vi "Poker Score.vi"(2 "Card Number":dbl) -> (0 "Poker Hands Score and Combination":T1(array[cluster]))   [LabVIEW 2014]
panel:
  in  "Pair's DBL":dbl
  in  "Pair's value":i32
  out "Score":dbl
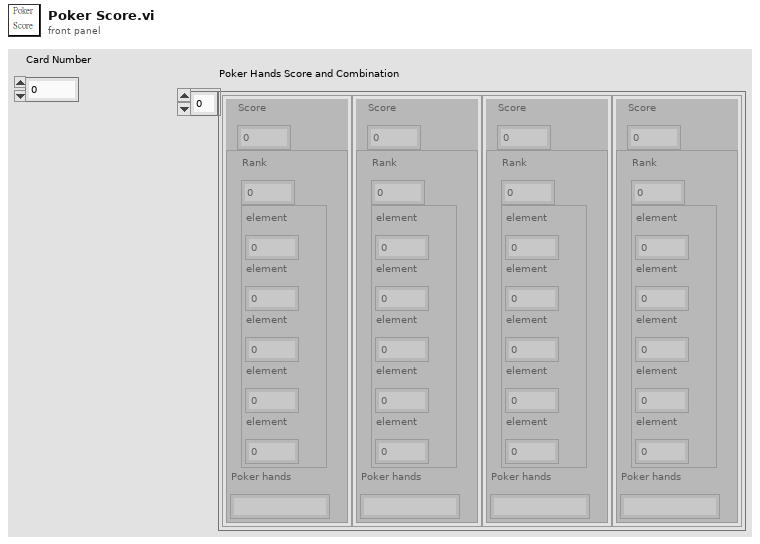
[diagram p1: front panel]
types:
  T1 = cluster{"Score":dbl, cluster{"Rank":i32, cluster{"element":dbl, "element":dbl, "element":dbl, "element":dbl, "element":dbl}, "Poker hands":string}}[]
  T2 = cluster{"Rank":i32, cluster{"element":dbl, "element":dbl, "element":dbl, "element":dbl, "element":dbl}, "Poker hands":string}[]
  T3 = cluster{"element":dbl, "element":dbl, "element":dbl, "element":dbl, "element":dbl}
  T4 = cluster{"Score":dbl, cluster{"Rank":i32, cluster{"element":dbl, "element":dbl, "element":dbl, "element":dbl, "element":dbl}, "Poker hands":string}}
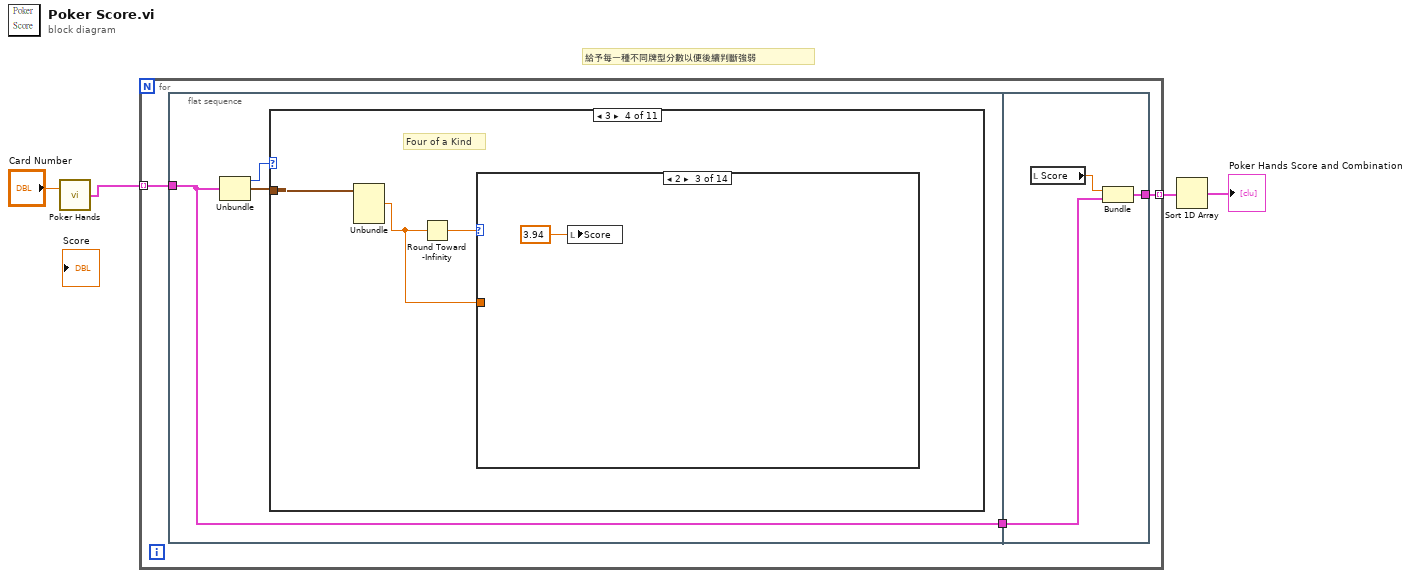
[diagram p0: block diagram]
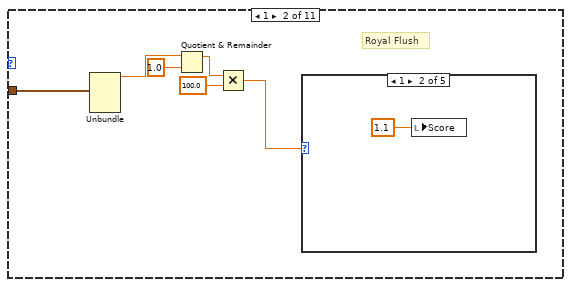
[diagram p3: hidden frame]
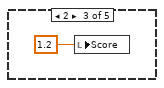
[diagram p5: hidden frame]
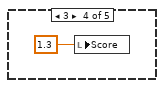
[diagram p6: hidden frame]
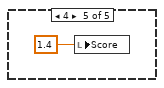
[diagram p7: hidden frame]
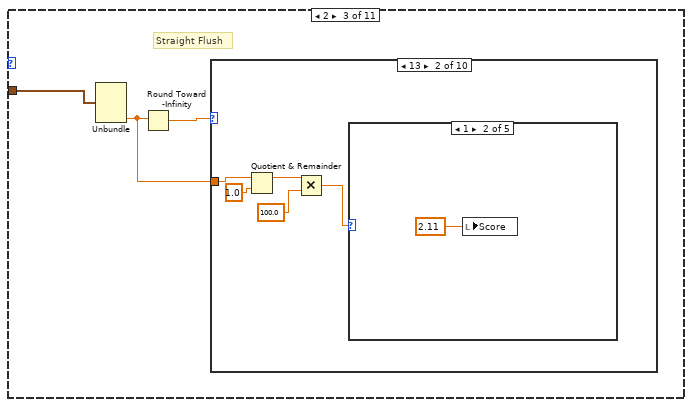
[diagram p8: hidden frame]
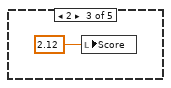
[diagram p11: hidden frame]
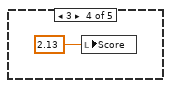
[diagram p12: hidden frame]
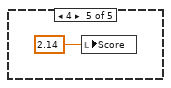
[diagram p13: hidden frame]
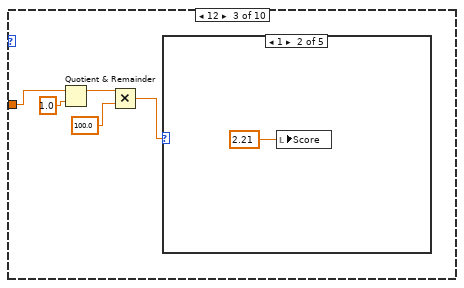
[diagram p14: hidden frame]
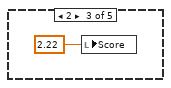
[diagram p16: hidden frame]
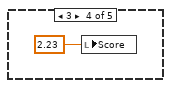
[diagram p17: hidden frame]
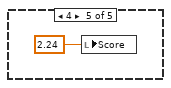
[diagram p18: hidden frame]
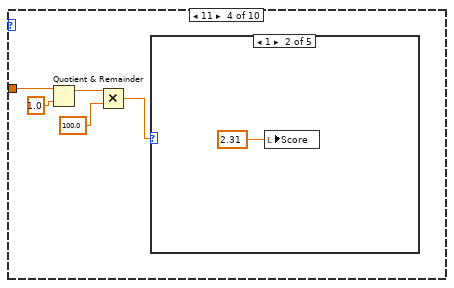
[diagram p19: hidden frame]
diagram:
  # "給予每一種不同牌型分數以便後續判斷強弱"
  n1 = call "Poker Hands.vi"("Card Number"="Card Number") -> ("Poker hands Rank and Combination"=w3:T2)  [unwired: 1 in]
  n2 = for {
    tunnel: w3 -> [w7] mode=indexing
    tunnel: [w5] -> w2 mode=indexing
    n3 = flat-sequence {
      tunnel: [w8] -> w6
      tunnel: w7 -> [w8]
      tunnel: w6 -> [w888]
      tunnel: [w887] -> w5
      frame #0 {
        n4 = Unbundle(w8) -> ("Rank"=w10:i32, w9:T3)  [unwired: 1 out]
        n5 = case shown="3" w10 {
          tunnel: w9 -> [_ w14 w23 w107 w123 w247 w322 w420 w555 w664 w808]
          frame 0, Default {
          }
          frame 1 {
            # "Royal Flush"
            n6 = Unbundle(w14) -> ("element"=w16:dbl)  [unwired: 4 out]
            n7 = Quotient & Remainder(x=w16, y=1.0) -> (x-y*floor(x/y)=w13:dbl)  [unwired: 1 out]
            n8 = Multiply(x=w13, y=100.0) -> (x*y=w11:dbl)
            n9 = case shown="1" w11 {
              frame 0, Default {
              }
              frame 1 {
                n10 = local write "Score"(1.1 ("Numeric")) -> ()
              }
              frame 2 {
                n11 = local write "Score"(1.2 ("Numeric")) -> ()
              }
              frame 3 {
                n12 = local write "Score"(1.3 ("Numeric")) -> ()
              }
              frame 4 {
                n13 = local write "Score"(1.4 ("Numeric")) -> ()
              }
            }
          }
          frame 2 {
            # "Straight Flush"
            n14 = Unbundle(w23) -> ("element"=w21:dbl)  [unwired: 4 out]
            n15 = Round Toward -Infinity(1:w21) -> (0:w22:dbl)
            n16 = case shown="13" w22 {
              tunnel: w21 -> [_ w28 w33 w42 w51 w60 w69 w78 w87 w96]
              frame 0, Default {
              }
              frame 13 {
                n17 = Quotient & Remainder(x=w28, y=1.0) -> (x-y*floor(x/y)=w26:dbl)  [unwired: 1 out]
                n18 = Multiply(x=w26, y=100.0) -> (x*y=w24:dbl)
                n19 = case shown="1" w24 {
                  frame 0, Default {
                  }
                  frame 1 {
                    n20 = local write "Score"(2.11 ("Numeric")) -> ()
                  }
                  frame 2 {
                    n21 = local write "Score"(2.12 ("Numeric")) -> ()
                  }
                  frame 3 {
                    n22 = local write "Score"(2.13 ("Numeric")) -> ()
                  }
                  frame 4 {
                    n23 = local write "Score"(2.14 ("Numeric")) -> ()
                  }
                }
              }
              frame 12 {
                n24 = Quotient & Remainder(x=w33, y=1.0) -> (x-y*floor(x/y)=w36:dbl)  [unwired: 1 out]
                n25 = Multiply(x=w36, y=100.0) -> (x*y=w34:dbl)
                n26 = case shown="1" w34 {
                  frame 0, Default {
                  }
                  frame 1 {
                    n27 = local write "Score"(2.21 ("Numeric")) -> ()
                  }
                  frame 2 {
                    n28 = local write "Score"(2.22 ("Numeric")) -> ()
                  }
                  frame 3 {
                    n29 = local write "Score"(2.23 ("Numeric")) -> ()
                  }
                  frame 4 {
                    n30 = local write "Score"(2.24 ("Numeric")) -> ()
                  }
                }
              }
              frame 11 {
                n31 = Quotient & Remainder(x=w42, y=1.0) -> (x-y*floor(x/y)=w45:dbl)  [unwired: 1 out]
                n32 = Multiply(x=w45, y=100.0) -> (x*y=w43:dbl)
                n33 = case shown="1" w43 {
                  frame 0, Default {
                  }
                  frame 1 {
                    n34 = local write "Score"(2.31 ("Numeric")) -> ()
                  }
                  frame 2 {
                    n35 = local write "Score"(2.32 ("Numeric")) -> ()
                  }
                  frame 3 {
                    n36 = local write "Score"(2.33 ("Numeric")) -> ()
                  }
                  frame 4 {
                    n37 = local write "Score"(2.34 ("Numeric")) -> ()
                  }
                }
              }
              frame 10 {
                n38 = Quotient & Remainder(x=w51, y=1.0) -> (x-y*floor(x/y)=w54:dbl)  [unwired: 1 out]
                n39 = Multiply(x=w54, y=100.0) -> (x*y=w52:dbl)
                n40 = case shown="1" w52 {
                  frame 0, Default {
                  }
                  frame 1 {
                    n41 = local write "Score"(2.41 ("Numeric")) -> ()
                  }
                  frame 2 {
                    n42 = local write "Score"(2.42 ("Numeric")) -> ()
                  }
                  frame 3 {
                    n43 = local write "Score"(2.43 ("Numeric")) -> ()
                  }
                  frame 4 {
                    n44 = local write "Score"(2.44 ("Numeric")) -> ()
                  }
                }
              }
              frame 9 {
                n45 = Quotient & Remainder(x=w60, y=1.0) -> (x-y*floor(x/y)=w63:dbl)  [unwired: 1 out]
                n46 = Multiply(x=w63, y=100.0) -> (x*y=w61:dbl)
                n47 = case shown="1" w61 {
                  frame 0, Default {
                  }
                  frame 1 {
                    n48 = local write "Score"(2.51 ("Numeric")) -> ()
                  }
                  frame 2 {
                    n49 = local write "Score"(2.52 ("Numeric")) -> ()
                  }
                  frame 3 {
                    n50 = local write "Score"(2.53 ("Numeric")) -> ()
                  }
                  frame 4 {
                    n51 = local write "Score"(2.54 ("Numeric")) -> ()
                  }
                }
              }
              frame 8 {
                n52 = Quotient & Remainder(x=w69, y=1.0) -> (x-y*floor(x/y)=w72:dbl)  [unwired: 1 out]
                n53 = Multiply(x=w72, y=100.0) -> (x*y=w70:dbl)
                n54 = case shown="1" w70 {
                  frame 0, Default {
                  }
                  frame 1 {
                    n55 = local write "Score"(2.61 ("Numeric")) -> ()
                  }
                  frame 2 {
                    n56 = local write "Score"(2.62 ("Numeric")) -> ()
                  }
                  frame 3 {
                    n57 = local write "Score"(2.63 ("Numeric")) -> ()
                  }
                  frame 4 {
                    n58 = local write "Score"(2.64 ("Numeric")) -> ()
                  }
                }
              }
              frame 7 {
                n59 = Quotient & Remainder(x=w78, y=1.0) -> (x-y*floor(x/y)=w81:dbl)  [unwired: 1 out]
                n60 = Multiply(x=w81, y=100.0) -> (x*y=w79:dbl)
                n61 = case shown="1" w79 {
                  frame 0, Default {
                  }
                  frame 1 {
                    n62 = local write "Score"(2.71 ("Numeric")) -> ()
                  }
                  frame 2 {
                    n63 = local write "Score"(2.72 ("Numeric")) -> ()
                  }
                  frame 3 {
                    n64 = local write "Score"(2.73 ("Numeric")) -> ()
                  }
                  frame 4 {
                    n65 = local write "Score"(2.74 ("Numeric")) -> ()
                  }
                }
              }
              frame 6 {
                n66 = Quotient & Remainder(x=w87, y=1.0) -> (x-y*floor(x/y)=w90:dbl)  [unwired: 1 out]
                n67 = Multiply(x=w90, y=100.0) -> (x*y=w88:dbl)
                n68 = case shown="1" w88 {
                  frame 0, Default {
                  }
                  frame 1 {
                    n69 = local write "Score"(2.81 ("Numeric")) -> ()
                  }
                  frame 2 {
                    n70 = local write "Score"(2.82 ("Numeric")) -> ()
                  }
                  frame 3 {
                    n71 = local write "Score"(2.83 ("Numeric")) -> ()
                  }
                  frame 4 {
                    n72 = local write "Score"(2.84 ("Numeric")) -> ()
                  }
                }
              }
              frame 5 {
                n73 = Quotient & Remainder(x=w96, y=1.0) -> (x-y*floor(x/y)=w99:dbl)  [unwired: 1 out]
                n74 = Multiply(x=w99, y=100.0) -> (x*y=w97:dbl)
                n75 = case shown="1" w97 {
                  frame 0, Default {
                  }
                  frame 1 {
                    n76 = local write "Score"(2.91 ("Numeric")) -> ()
                  }
                  frame 2 {
                    n77 = local write "Score"(2.92 ("Numeric")) -> ()
                  }
                  frame 3 {
                    n78 = local write "Score"(2.93 ("Numeric")) -> ()
                  }
                  frame 4 {
                    n79 = local write "Score"(2.94 ("Numeric")) -> ()
                  }
                }
              }
            }
          }
          frame 3 {
            # "Four of a Kind"
            n80 = Unbundle(w107) -> ("element"=w105:dbl)  [unwired: 4 out]
            n81 = Round Toward -Infinity(1:w105) -> (0:w106:dbl)
            n82 = case shown="2" w106 {
              tunnel: w105 -> [_ _ _ _ _ _ _ _ _ _ _ _ _ _]
              frame 0, Default {
              }
              frame 1 {
                n83 = local write "Score"(3.1 ("Numeric")) -> ()
              }
              frame 2 {
                n84 = local write "Score"(3.94 ("Numeric")) -> ()
              }
              frame 3 {
                n85 = local write "Score"(3.93 ("Numeric")) -> ()
              }
              frame 4 {
                n86 = local write "Score"(3.92 ("Numeric")) -> ()
              }
              frame 5 {
                n87 = local write "Score"(3.91 ("Numeric")) -> ()
              }
              frame 6 {
                n88 = local write "Score"(3.9 ("Numeric")) -> ()
              }
              frame 7 {
                n89 = local write "Score"(3.8 ("Numeric")) -> ()
              }
              frame 8 {
                n90 = local write "Score"(3.7 ("Numeric")) -> ()
              }
              frame 9 {
                n91 = local write "Score"(3.6 ("Numeric")) -> ()
              }
              frame 10 {
                n92 = local write "Score"(3.5 ("Numeric")) -> ()
              }
              frame 11 {
                n93 = local write "Score"(3.4 ("Numeric")) -> ()
              }
              frame 12 {
                n94 = local write "Score"(3.3 ("Numeric")) -> ()
              }
              frame 13 {
                n95 = local write "Score"(3.2 ("Numeric")) -> ()
              }
            }
          }
          frame 4 {
            # "Full House"
            n96 = Unbundle(w123) -> ("element"=w121:dbl)  [unwired: 4 out]
            n97 = Round Toward -Infinity(1:w121) -> (0:w122:dbl)
            n98 = case shown="1" w122 {
              tunnel: w121 -> [_ w124 w133 w142 w151 w160 w169 w178 w187 w196 w205 w214 w223 w232]
              frame 0, Default {
              }
              frame 1 {
                n99 = Quotient & Remainder(x=w124, y=1.0) -> (x-y*floor(x/y)=w127:dbl)  [unwired: 1 out]
                n100 = Multiply(x=w127, y=100.0) -> (x*y=w125:dbl)
                n101 = case shown="1" w125 {
                  frame 0, Default {
                  }
                  frame 1 {
                    n102 = local write "Score"(4.11 ("Numeric")) -> ()
                  }
                  frame 2 {
                    n103 = local write "Score"(4.12 ("Numeric")) -> ()
                  }
                  frame 3 {
                    n104 = local write "Score"(4.13 ("Numeric")) -> ()
                  }
                  frame 4 {
                    n105 = local write "Score"(4.14 ("Numeric")) -> ()
                  }
                }
              }
              frame 2 {
                n106 = Quotient & Remainder(x=w133, y=1.0) -> (x-y*floor(x/y)=w136:dbl)  [unwired: 1 out]
                n107 = Multiply(x=w136, y=100.0) -> (x*y=w134:dbl)
                n108 = case shown="4" w134 {
                  frame 0, Default {
                  }
                  frame 1 {
                    n109 = local write "Score"(4.981 ("Numeric")) -> ()
                  }
                  frame 2 {
                    n110 = local write "Score"(4.982 ("Numeric")) -> ()
                  }
                  frame 3 {
                    n111 = local write "Score"(4.983 ("Numeric")) -> ()
                  }
                  frame 4 {
                    n112 = local write "Score"(4.984 ("Numeric")) -> ()
                  }
                }
              }
              frame 3 {
                n113 = Quotient & Remainder(x=w142, y=1.0) -> (x-y*floor(x/y)=w145:dbl)  [unwired: 1 out]
                n114 = Multiply(x=w145, y=100.0) -> (x*y=w143:dbl)
                n115 = case shown="4" w143 {
                  frame 0, Default {
                  }
                  frame 1 {
                    n116 = local write "Score"(4.971 ("Numeric")) -> ()
                  }
                  frame 2 {
                    n117 = local write "Score"(4.972 ("Numeric")) -> ()
                  }
                  frame 3 {
                    n118 = local write "Score"(4.973 ("Numeric")) -> ()
                  }
                  frame 4 {
                    n119 = local write "Score"(4.974 ("Numeric")) -> ()
                  }
                }
              }
              frame 4 {
                n120 = Quotient & Remainder(x=w151, y=1.0) -> (x-y*floor(x/y)=w154:dbl)  [unwired: 1 out]
                n121 = Multiply(x=w154, y=100.0) -> (x*y=w152:dbl)
                n122 = case shown="3" w152 {
                  frame 0, Default {
                  }
                  frame 1 {
                    n123 = local write "Score"(4.961 ("Numeric")) -> ()
                  }
                  frame 2 {
                    n124 = local write "Score"(4.962 ("Numeric")) -> ()
                  }
                  frame 3 {
                    n125 = local write "Score"(4.963 ("Numeric")) -> ()
                  }
                  frame 4 {
                    n126 = local write "Score"(4.964 ("Numeric")) -> ()
                  }
                }
              }
              frame 5 {
                n127 = Quotient & Remainder(x=w160, y=1.0) -> (x-y*floor(x/y)=w163:dbl)  [unwired: 1 out]
                n128 = Multiply(x=w163, y=100.0) -> (x*y=w161:dbl)
                n129 = case shown="4" w161 {
                  frame 0, Default {
                  }
                  frame 1 {
                    n130 = local write "Score"(4.951 ("Numeric")) -> ()
                  }
                  frame 2 {
                    n131 = local write "Score"(4.952 ("Numeric")) -> ()
                  }
                  frame 3 {
                    n132 = local write "Score"(4.953 ("Numeric")) -> ()
                  }
                  frame 4 {
                    n133 = local write "Score"(4.954 ("Numeric")) -> ()
                  }
                }
              }
              frame 6 {
                n134 = Quotient & Remainder(x=w169, y=1.0) -> (x-y*floor(x/y)=w172:dbl)  [unwired: 1 out]
                n135 = Multiply(x=w172, y=100.0) -> (x*y=w170:dbl)
                n136 = case shown="4" w170 {
                  frame 0, Default {
                  }
                  frame 1 {
                    n137 = local write "Score"(4.91 ("Numeric")) -> ()
                  }
                  frame 2 {
                    n138 = local write "Score"(4.92 ("Numeric")) -> ()
                  }
                  frame 3 {
                    n139 = local write "Score"(4.93 ("Numeric")) -> ()
                  }
                  frame 4 {
                    n140 = local write "Score"(4.94 ("Numeric")) -> ()
                  }
                }
              }
              frame 7 {
                n141 = Quotient & Remainder(x=w178, y=1.0) -> (x-y*floor(x/y)=w181:dbl)  [unwired: 1 out]
                n142 = Multiply(x=w181, y=100.0) -> (x*y=w179:dbl)
                n143 = case shown="4" w179 {
                  frame 0, Default {
                  }
                  frame 1 {
                    n144 = local write "Score"(4.81 ("Numeric")) -> ()
                  }
                  frame 2 {
                    n145 = local write "Score"(4.82 ("Numeric")) -> ()
                  }
                  frame 3 {
                    n146 = local write "Score"(4.83 ("Numeric")) -> ()
                  }
                  frame 4 {
                    n147 = local write "Score"(4.84 ("Numeric")) -> ()
                  }
                }
              }
              frame 8 {
                n148 = Quotient & Remainder(x=w187, y=1.0) -> (x-y*floor(x/y)=w190:dbl)  [unwired: 1 out]
                n149 = Multiply(x=w190, y=100.0) -> (x*y=w188:dbl)
                n150 = case shown="3" w188 {
                  frame 0, Default {
                  }
                  frame 1 {
                    n151 = local write "Score"(4.71 ("Numeric")) -> ()
                  }
                  frame 2 {
                    n152 = local write "Score"(4.72 ("Numeric")) -> ()
                  }
                  frame 3 {
                    n153 = local write "Score"(4.73 ("Numeric")) -> ()
                  }
                  frame 4 {
                    n154 = local write "Score"(4.74 ("Numeric")) -> ()
                  }
                }
              }
              frame 9 {
                n155 = Quotient & Remainder(x=w196, y=1.0) -> (x-y*floor(x/y)=w199:dbl)  [unwired: 1 out]
                n156 = Multiply(x=w199, y=100.0) -> (x*y=w197:dbl)
                n157 = case shown="4" w197 {
                  frame 0, Default {
                  }
                  frame 1 {
                    n158 = local write "Score"(4.61 ("Numeric")) -> ()
                  }
                  frame 2 {
                    n159 = local write "Score"(4.62 ("Numeric")) -> ()
                  }
                  frame 3 {
                    n160 = local write "Score"(4.63 ("Numeric")) -> ()
                  }
                  frame 4 {
                    n161 = local write "Score"(4.64 ("Numeric")) -> ()
                  }
                }
              }
              frame 10 {
                n162 = Quotient & Remainder(x=w205, y=1.0) -> (x-y*floor(x/y)=w208:dbl)  [unwired: 1 out]
                n163 = Multiply(x=w208, y=100.0) -> (x*y=w206:dbl)
                n164 = case shown="1" w206 {
                  frame 0, Default {
                  }
                  frame 1 {
                    n165 = local write "Score"(4.51 ("Numeric")) -> ()
                  }
                  frame 2 {
                    n166 = local write "Score"(4.52 ("Numeric")) -> ()
                  }
                  frame 3 {
                    n167 = local write "Score"(4.53 ("Numeric")) -> ()
                  }
                  frame 4 {
                    n168 = local write "Score"(4.54 ("Numeric")) -> ()
                  }
                }
              }
              frame 11 {
                n169 = Quotient & Remainder(x=w214, y=1.0) -> (x-y*floor(x/y)=w217:dbl)  [unwired: 1 out]
                n170 = Multiply(x=w217, y=100.0) -> (x*y=w215:dbl)
                n171 = case shown="1" w215 {
                  frame 0, Default {
                  }
                  frame 1 {
                    n172 = local write "Score"(4.41 ("Numeric")) -> ()
                  }
                  frame 2 {
                    n173 = local write "Score"(4.42 ("Numeric")) -> ()
                  }
                  frame 3 {
                    n174 = local write "Score"(4.43 ("Numeric")) -> ()
                  }
                  frame 4 {
                    n175 = local write "Score"(4.44 ("Numeric")) -> ()
                  }
                }
              }
              frame 12 {
                n176 = Quotient & Remainder(x=w223, y=1.0) -> (x-y*floor(x/y)=w226:dbl)  [unwired: 1 out]
                n177 = Multiply(x=w226, y=100.0) -> (x*y=w224:dbl)
                n178 = case shown="2" w224 {
                  frame 0, Default {
                  }
                  frame 1 {
                    n179 = local write "Score"(4.31 ("Numeric")) -> ()
                  }
                  frame 2 {
                    n180 = local write "Score"(4.32 ("Numeric")) -> ()
                  }
                  frame 3 {
                    n181 = local write "Score"(4.33 ("Numeric")) -> ()
                  }
                  frame 4 {
                    n182 = local write "Score"(4.34 ("Numeric")) -> ()
                  }
                }
              }
              frame 13 {
                n183 = Quotient & Remainder(x=w232, y=1.0) -> (x-y*floor(x/y)=w235:dbl)  [unwired: 1 out]
                n184 = Multiply(x=w235, y=100.0) -> (x*y=w233:dbl)
                n185 = case shown="4" w233 {
                  frame 0, Default {
                  }
                  frame 1 {
                    n186 = local write "Score"(4.21 ("Numeric")) -> ()
                  }
                  frame 2 {
                    n187 = local write "Score"(4.22 ("Numeric")) -> ()
                  }
                  frame 3 {
                    n188 = local write "Score"(4.23 ("Numeric")) -> ()
                  }
                  frame 4 {
                    n189 = local write "Score"(4.24 ("Numeric")) -> ()
                  }
                }
              }
            }
          }
          frame 5 {
            # "Flush"
            n190 = Unbundle(w247) -> ("element"=w242:dbl, "element"=w241:dbl)  [unwired: 3 out]
            n191 = Round Toward -Infinity(1:w242) -> (0:w246:dbl)
            n192 = Round Toward -Infinity(1:w241) -> (0:w243:dbl)
            n193 = Equal?(x=w246, y=1.0) -> (x = y?=w245:bool)
            n194 = case shown="7" w243 {
              tunnel: w241 -> [_ w248 w257 w266 w275 w284 w293 w302]
              frame 0, Default {
              }
              frame 7 {
                n195 = Quotient & Remainder(x=w248, y=1.0) -> (x-y*floor(x/y)=w251:dbl)  [unwired: 1 out]
                n196 = Multiply(x=w251, y=100.0) -> (x*y=w249:dbl)
                n197 = case shown="4" w249 {
                  frame 0, Default {
                  }
                  frame 1 {
                    n198 = local write "Score"(5.81 ("Numeric")) -> ()
                  }
                  frame 2 {
                    n199 = local write "Score"(5.82 ("Numeric")) -> ()
                  }
                  frame 3 {
                    n200 = local write "Score"(5.83 ("Numeric")) -> ()
                  }
                  frame 4 {
                    n201 = local write "Score"(5.84 ("Numeric")) -> ()
                  }
                }
              }
              frame 8 {
                n202 = Quotient & Remainder(x=w257, y=1.0) -> (x-y*floor(x/y)=w260:dbl)  [unwired: 1 out]
                n203 = Multiply(x=w260, y=100.0) -> (x*y=w258:dbl)
                n204 = case shown="4" w258 {
                  frame 0, Default {
                  }
                  frame 1 {
                    n205 = local write "Score"(5.71 ("Numeric")) -> ()
                  }
                  frame 2 {
                    n206 = local write "Score"(5.72 ("Numeric")) -> ()
                  }
                  frame 3 {
                    n207 = local write "Score"(5.73 ("Numeric")) -> ()
                  }
                  frame 4 {
                    n208 = local write "Score"(5.74 ("Numeric")) -> ()
                  }
                }
              }
              frame 9 {
                n209 = Quotient & Remainder(x=w266, y=1.0) -> (x-y*floor(x/y)=w269:dbl)  [unwired: 1 out]
                n210 = Multiply(x=w269, y=100.0) -> (x*y=w267:dbl)
                n211 = case shown="1" w267 {
                  frame 0, Default {
                  }
                  frame 1 {
                    n212 = local write "Score"(5.61 ("Numeric")) -> ()
                  }
                  frame 2 {
                    n213 = local write "Score"(5.62 ("Numeric")) -> ()
                  }
                  frame 3 {
                    n214 = local write "Score"(5.63 ("Numeric")) -> ()
                  }
                  frame 4 {
                    n215 = local write "Score"(5.64 ("Numeric")) -> ()
                  }
                }
              }
              frame 10 {
                n216 = Quotient & Remainder(x=w275, y=1.0) -> (x-y*floor(x/y)=w278:dbl)  [unwired: 1 out]
                n217 = Multiply(x=w278, y=100.0) -> (x*y=w276:dbl)
                n218 = case shown="4" w276 {
                  frame 0, Default {
                  }
                  frame 1 {
                    n219 = local write "Score"(5.51 ("Numeric")) -> ()
                  }
                  frame 2 {
                    n220 = local write "Score"(5.52 ("Numeric")) -> ()
                  }
                  frame 3 {
                    n221 = local write "Score"(5.53 ("Numeric")) -> ()
                  }
                  frame 4 {
                    n222 = local write "Score"(5.54 ("Numeric")) -> ()
                  }
                }
              }
              frame 11 {
                n223 = Quotient & Remainder(x=w284, y=1.0) -> (x-y*floor(x/y)=w287:dbl)  [unwired: 1 out]
                n224 = Multiply(x=w287, y=100.0) -> (x*y=w285:dbl)
                n225 = case shown="4" w285 {
                  frame 0, Default {
                  }
                  frame 1 {
                    n226 = local write "Score"(5.41 ("Numeric")) -> ()
                  }
                  frame 2 {
                    n227 = local write "Score"(5.42 ("Numeric")) -> ()
                  }
                  frame 3 {
                    n228 = local write "Score"(5.43 ("Numeric")) -> ()
                  }
                  frame 4 {
                    n229 = local write "Score"(5.44 ("Numeric")) -> ()
                  }
                }
              }
              frame 12 {
                n230 = Quotient & Remainder(x=w293, y=1.0) -> (x-y*floor(x/y)=w296:dbl)  [unwired: 1 out]
                n231 = Multiply(x=w296, y=100.0) -> (x*y=w294:dbl)
                n232 = case shown="4" w294 {
                  frame 0, Default {
                  }
                  frame 1 {
                    n233 = local write "Score"(5.31 ("Numeric")) -> ()
                  }
                  frame 2 {
                    n234 = local write "Score"(5.32 ("Numeric")) -> ()
                  }
                  frame 3 {
                    n235 = local write "Score"(5.33 ("Numeric")) -> ()
                  }
                  frame 4 {
                    n236 = local write "Score"(5.34 ("Numeric")) -> ()
                  }
                }
              }
              frame 13 {
                n237 = Quotient & Remainder(x=w302, y=1.0) -> (x-y*floor(x/y)=w305:dbl)  [unwired: 1 out]
                n238 = Multiply(x=w305, y=100.0) -> (x*y=w303:dbl)
                n239 = case shown="4" w303 {
                  frame 0, Default {
                  }
                  frame 1 {
                    n240 = local write "Score"(5.21 ("Numeric")) -> ()
                  }
                  frame 2 {
                    n241 = local write "Score"(5.22 ("Numeric")) -> ()
                  }
                  frame 3 {
                    n242 = local write "Score"(5.23 ("Numeric")) -> ()
                  }
                  frame 4 {
                    n243 = local write "Score"(5.24 ("Numeric")) -> ()
                  }
                }
              }
            }
            n244 = case shown="True" w245 {
              tunnel: w242 -> [_ w311]
              frame False {
              }
              frame True {
                n245 = Quotient & Remainder(x=w311, y=1.0) -> (x-y*floor(x/y)=w314:dbl)  [unwired: 1 out]
                n246 = Multiply(x=w314, y=100.0) -> (x*y=w312:dbl)
                n247 = case shown="1" w312 {
                  frame 0, Default {
                  }
                  frame 1 {
                    n248 = local write "Score"(5.11 ("Numeric")) -> ()
                  }
                  frame 2 {
                    n249 = local write "Score"(5.12 ("Numeric")) -> ()
                  }
                  frame 3 {
                    n250 = local write "Score"(5.13 ("Numeric")) -> ()
                  }
                  frame 4 {
                    n251 = local write "Score"(5.14 ("Numeric")) -> ()
                  }
                }
              }
            }
          }
          frame 6 {
            # "Straight"
            n252 = Unbundle(w322) -> ("element"=w320:dbl, "element"=w323:dbl)  [unwired: 3 out]
            n253 = Round Toward -Infinity(1:w323) -> (0:w324:dbl)
            n254 = Round Toward -Infinity(1:w320) -> (0:w321:dbl)
            n255 = case shown="13" w324 {
              tunnel: w323 -> [_ w325 w348 w357 w366 w375 w384 w393 w402 w411]
              tunnel: w321 -> [_ w329 _ _ _ _ _ _ _ _]
              tunnel: w320 -> [_ w326 _ _ _ _ _ _ _ _]
              frame 0, Default {
              }
              frame 13 {
                n256 = Equal?(x=w329, y=1.0) -> (x = y?=w327:bool)
                n257 = case shown="False" w327 {
                  tunnel: w326 -> [_ w339]
                  tunnel: w325 -> [w330 _]
                  frame False {
                    n258 = Quotient & Remainder(x=w330, y=1.0) -> (x-y*floor(x/y)=w333:dbl)  [unwired: 1 out]
                    n259 = Multiply(x=w333, y=100.0) -> (x*y=w331:dbl)
                    n260 = case shown="4" w331 {
                      frame 0, Default {
                      }
                      frame 1 {
                        n261 = local write "Score"(6.11 ("Numeric")) -> ()
                      }
                      frame 2 {
                        n262 = local write "Score"(6.12 ("Numeric")) -> ()
                      }
                      frame 3 {
                        n263 = local write "Score"(6.13 ("Numeric")) -> ()
                      }
                      frame 4 {
                        n264 = local write "Score"(6.14 ("Numeric")) -> ()
                      }
                    }
                  }
                  frame True {
                    n265 = Quotient & Remainder(x=w339, y=1.0) -> (x-y*floor(x/y)=w342:dbl)  [unwired: 1 out]
                    n266 = Multiply(x=w342, y=100.0) -> (x*y=w340:dbl)
                    n267 = case shown="1" w340 {
                      frame 0, Default {
                      }
                      frame 1 {
                        n268 = local write "Score"(6.01 ("Numeric")) -> ()
                      }
                      frame 2 {
                        n269 = local write "Score"(6.02 ("Numeric")) -> ()
                      }
                      frame 3 {
                        n270 = local write "Score"(6.03 ("Numeric")) -> ()
                      }
                      frame 4 {
                        n271 = local write "Score"(6.04 ("Numeric")) -> ()
                      }
                    }
                  }
                }
              }
              frame 12 {
                n272 = Quotient & Remainder(x=w348, y=1.0) -> (x-y*floor(x/y)=w351:dbl)  [unwired: 1 out]
                n273 = Multiply(x=w351, y=100.0) -> (x*y=w349:dbl)
                n274 = case shown="4" w349 {
                  frame 0, Default {
                  }
                  frame 1 {
                    n275 = local write "Score"(6.21 ("Numeric")) -> ()
                  }
                  frame 2 {
                    n276 = local write "Score"(6.22 ("Numeric")) -> ()
                  }
                  frame 3 {
                    n277 = local write "Score"(6.23 ("Numeric")) -> ()
                  }
                  frame 4 {
                    n278 = local write "Score"(6.24 ("Numeric")) -> ()
                  }
                }
              }
              frame 11 {
                n279 = Quotient & Remainder(x=w357, y=1.0) -> (x-y*floor(x/y)=w360:dbl)  [unwired: 1 out]
                n280 = Multiply(x=w360, y=100.0) -> (x*y=w358:dbl)
                n281 = case shown="1" w358 {
                  frame 0, Default {
                  }
                  frame 1 {
                    n282 = local write "Score"(6.31 ("Numeric")) -> ()
                  }
                  frame 2 {
                    n283 = local write "Score"(6.32 ("Numeric")) -> ()
                  }
                  frame 3 {
                    n284 = local write "Score"(6.33 ("Numeric")) -> ()
                  }
                  frame 4 {
                    n285 = local write "Score"(6.34 ("Numeric")) -> ()
                  }
                }
              }
              frame 10 {
                n286 = Quotient & Remainder(x=w366, y=1.0) -> (x-y*floor(x/y)=w369:dbl)  [unwired: 1 out]
                n287 = Multiply(x=w369, y=100.0) -> (x*y=w367:dbl)
                n288 = case shown="4" w367 {
                  frame 0, Default {
                  }
                  frame 1 {
                    n289 = local write "Score"(6.41 ("Numeric")) -> ()
                  }
                  frame 2 {
                    n290 = local write "Score"(6.42 ("Numeric")) -> ()
                  }
                  frame 3 {
                    n291 = local write "Score"(6.43 ("Numeric")) -> ()
                  }
                  frame 4 {
                    n292 = local write "Score"(6.44 ("Numeric")) -> ()
                  }
                }
              }
              frame 9 {
                n293 = Quotient & Remainder(x=w375, y=1.0) -> (x-y*floor(x/y)=w378:dbl)  [unwired: 1 out]
                n294 = Multiply(x=w378, y=100.0) -> (x*y=w376:dbl)
                n295 = case shown="4" w376 {
                  frame 0, Default {
                  }
                  frame 1 {
                    n296 = local write "Score"(6.51 ("Numeric")) -> ()
                  }
                  frame 2 {
                    n297 = local write "Score"(6.52 ("Numeric")) -> ()
                  }
                  frame 3 {
                    n298 = local write "Score"(6.53 ("Numeric")) -> ()
                  }
                  frame 4 {
                    n299 = local write "Score"(6.54 ("Numeric")) -> ()
                  }
                }
              }
              frame 8 {
                n300 = Quotient & Remainder(x=w384, y=1.0) -> (x-y*floor(x/y)=w387:dbl)  [unwired: 1 out]
                n301 = Multiply(x=w387, y=100.0) -> (x*y=w385:dbl)
                n302 = case shown="4" w385 {
                  frame 0, Default {
                  }
                  frame 1 {
                    n303 = local write "Score"(6.61 ("Numeric")) -> ()
                  }
                  frame 2 {
                    n304 = local write "Score"(6.62 ("Numeric")) -> ()
                  }
                  frame 3 {
                    n305 = local write "Score"(6.63 ("Numeric")) -> ()
                  }
                  frame 4 {
                    n306 = local write "Score"(6.64 ("Numeric")) -> ()
                  }
                }
              }
              frame 7 {
                n307 = Quotient & Remainder(x=w393, y=1.0) -> (x-y*floor(x/y)=w396:dbl)  [unwired: 1 out]
                n308 = Multiply(x=w396, y=100.0) -> (x*y=w394:dbl)
                n309 = case shown="4" w394 {
                  frame 0, Default {
                  }
                  frame 1 {
                    n310 = local write "Score"(6.71 ("Numeric")) -> ()
                  }
                  frame 2 {
                    n311 = local write "Score"(6.72 ("Numeric")) -> ()
                  }
                  frame 3 {
                    n312 = local write "Score"(6.73 ("Numeric")) -> ()
                  }
                  frame 4 {
                    n313 = local write "Score"(6.74 ("Numeric")) -> ()
                  }
                }
              }
              frame 6 {
                n314 = Quotient & Remainder(x=w402, y=1.0) -> (x-y*floor(x/y)=w405:dbl)  [unwired: 1 out]
                n315 = Multiply(x=w405, y=100.0) -> (x*y=w403:dbl)
                n316 = case shown="4" w403 {
                  frame 0, Default {
                  }
                  frame 1 {
                    n317 = local write "Score"(6.81 ("Numeric")) -> ()
                  }
                  frame 2 {
                    n318 = local write "Score"(6.82 ("Numeric")) -> ()
                  }
                  frame 3 {
                    n319 = local write "Score"(6.83 ("Numeric")) -> ()
                  }
                  frame 4 {
                    n320 = local write "Score"(6.84 ("Numeric")) -> ()
                  }
                }
              }
              frame 5 {
                n321 = Quotient & Remainder(x=w411, y=1.0) -> (x-y*floor(x/y)=w414:dbl)  [unwired: 1 out]
                n322 = Multiply(x=w414, y=100.0) -> (x*y=w412:dbl)
                n323 = case shown="4" w412 {
                  frame 0, Default {
                  }
                  frame 1 {
                    n324 = local write "Score"(6.91 ("Numeric")) -> ()
                  }
                  frame 2 {
                    n325 = local write "Score"(6.92 ("Numeric")) -> ()
                  }
                  frame 3 {
                    n326 = local write "Score"(6.93 ("Numeric")) -> ()
                  }
                  frame 4 {
                    n327 = local write "Score"(6.94 ("Numeric")) -> ()
                  }
                }
              }
            }
          }
          frame 7 {
            # "Three of a kind"
            n328 = Unbundle(w420) -> ("element"=w421:dbl)  [unwired: 4 out]
            n329 = Round Toward -Infinity(1:w421) -> (0:w422:dbl)
            n330 = case shown="1" w422 {
              tunnel: w421 -> [_ w423 w432 w441 w450 w459 w468 w477 w486 w495 w504 w513 w522 w531]
              frame 0, Default {
              }
              frame 1 {
                n331 = Quotient & Remainder(x=w423, y=1.0) -> (x-y*floor(x/y)=w426:dbl)  [unwired: 1 out]
                n332 = Multiply(x=w426, y=100.0) -> (x*y=w424:dbl)
                n333 = case shown="4" w424 {
                  frame 0, Default {
                  }
                  frame 1 {
                    n334 = local write "Score"(7.11 ("Numeric")) -> ()
                  }
                  frame 2 {
                    n335 = local write "Score"(7.12 ("Numeric")) -> ()
                  }
                  frame 3 {
                    n336 = local write "Score"(7.13 ("Numeric")) -> ()
                  }
                  frame 4 {
                    n337 = local write "Score"(7.14 ("Numeric")) -> ()
                  }
                }
              }
              frame 2 {
                n338 = Quotient & Remainder(x=w432, y=1.0) -> (x-y*floor(x/y)=w435:dbl)  [unwired: 1 out]
                n339 = Multiply(x=w435, y=100.0) -> (x*y=w433:dbl)
                n340 = case shown="4" w433 {
                  frame 0, Default {
                  }
                  frame 1 {
                    n341 = local write "Score"(7.981 ("Numeric")) -> ()
                  }
                  frame 2 {
                    n342 = local write "Score"(7.982 ("Numeric")) -> ()
                  }
                  frame 3 {
                    n343 = local write "Score"(7.983 ("Numeric")) -> ()
                  }
                  frame 4 {
                    n344 = local write "Score"(7.984 ("Numeric")) -> ()
                  }
                }
              }
              frame 3 {
                n345 = Quotient & Remainder(x=w441, y=1.0) -> (x-y*floor(x/y)=w444:dbl)  [unwired: 1 out]
                n346 = Multiply(x=w444, y=100.0) -> (x*y=w442:dbl)
                n347 = case shown="4" w442 {
                  frame 0, Default {
                  }
                  frame 1 {
                    n348 = local write "Score"(7.971 ("Numeric")) -> ()
                  }
                  frame 2 {
                    n349 = local write "Score"(7.972 ("Numeric")) -> ()
                  }
                  frame 3 {
                    n350 = local write "Score"(7.973 ("Numeric")) -> ()
                  }
                  frame 4 {
                    n351 = local write "Score"(7.974 ("Numeric")) -> ()
                  }
                }
              }
              frame 4 {
                n352 = Quotient & Remainder(x=w450, y=1.0) -> (x-y*floor(x/y)=w453:dbl)  [unwired: 1 out]
                n353 = Multiply(x=w453, y=100.0) -> (x*y=w451:dbl)
                n354 = case shown="4" w451 {
                  frame 0, Default {
                  }
                  frame 1 {
                    n355 = local write "Score"(7.961 ("Numeric")) -> ()
                  }
                  frame 2 {
                    n356 = local write "Score"(7.962 ("Numeric")) -> ()
                  }
                  frame 3 {
                    n357 = local write "Score"(7.963 ("Numeric")) -> ()
                  }
                  frame 4 {
                    n358 = local write "Score"(7.964 ("Numeric")) -> ()
                  }
                }
              }
              frame 5 {
                n359 = Quotient & Remainder(x=w459, y=1.0) -> (x-y*floor(x/y)=w462:dbl)  [unwired: 1 out]
                n360 = Multiply(x=w462, y=100.0) -> (x*y=w460:dbl)
                n361 = case shown="4" w460 {
                  frame 0, Default {
                  }
                  frame 1 {
                    n362 = local write "Score"(7.951 ("Numeric")) -> ()
                  }
                  frame 2 {
                    n363 = local write "Score"(7.952 ("Numeric")) -> ()
                  }
                  frame 3 {
                    n364 = local write "Score"(7.953 ("Numeric")) -> ()
                  }
                  frame 4 {
                    n365 = local write "Score"(7.954 ("Numeric")) -> ()
                  }
                }
              }
              frame 6 {
                n366 = Quotient & Remainder(x=w468, y=1.0) -> (x-y*floor(x/y)=w471:dbl)  [unwired: 1 out]
                n367 = Multiply(x=w471, y=100.0) -> (x*y=w469:dbl)
                n368 = case shown="4" w469 {
                  frame 0, Default {
                  }
                  frame 1 {
                    n369 = local write "Score"(7.91 ("Numeric")) -> ()
                  }
                  frame 2 {
                    n370 = local write "Score"(7.92 ("Numeric")) -> ()
                  }
                  frame 3 {
                    n371 = local write "Score"(7.93 ("Numeric")) -> ()
                  }
                  frame 4 {
                    n372 = local write "Score"(7.94 ("Numeric")) -> ()
                  }
                }
              }
              frame 7 {
                n373 = Quotient & Remainder(x=w477, y=1.0) -> (x-y*floor(x/y)=w480:dbl)  [unwired: 1 out]
                n374 = Multiply(x=w480, y=100.0) -> (x*y=w478:dbl)
                n375 = case shown="4" w478 {
                  frame 0, Default {
                  }
                  frame 1 {
                    n376 = local write "Score"(7.81 ("Numeric")) -> ()
                  }
                  frame 2 {
                    n377 = local write "Score"(7.82 ("Numeric")) -> ()
                  }
                  frame 3 {
                    n378 = local write "Score"(7.83 ("Numeric")) -> ()
                  }
                  frame 4 {
                    n379 = local write "Score"(7.84 ("Numeric")) -> ()
                  }
                }
              }
              frame 8 {
                n380 = Quotient & Remainder(x=w486, y=1.0) -> (x-y*floor(x/y)=w489:dbl)  [unwired: 1 out]
                n381 = Multiply(x=w489, y=100.0) -> (x*y=w487:dbl)
                n382 = case shown="4" w487 {
                  frame 0, Default {
                  }
                  frame 1 {
                    n383 = local write "Score"(7.71 ("Numeric")) -> ()
                  }
                  frame 2 {
                    n384 = local write "Score"(7.72 ("Numeric")) -> ()
                  }
                  frame 3 {
                    n385 = local write "Score"(7.73 ("Numeric")) -> ()
                  }
                  frame 4 {
                    n386 = local write "Score"(7.74 ("Numeric")) -> ()
                  }
                }
              }
              frame 9 {
                n387 = Quotient & Remainder(x=w495, y=1.0) -> (x-y*floor(x/y)=w498:dbl)  [unwired: 1 out]
                n388 = Multiply(x=w498, y=100.0) -> (x*y=w496:dbl)
                n389 = case shown="3" w496 {
                  frame 0, Default {
                  }
                  frame 1 {
                    n390 = local write "Score"(7.61 ("Numeric")) -> ()
                  }
                  frame 2 {
                    n391 = local write "Score"(7.62 ("Numeric")) -> ()
                  }
                  frame 3 {
                    n392 = local write "Score"(7.63 ("Numeric")) -> ()
                  }
                  frame 4 {
                    n393 = local write "Score"(7.64 ("Numeric")) -> ()
                  }
                }
              }
              frame 10 {
                n394 = Quotient & Remainder(x=w504, y=1.0) -> (x-y*floor(x/y)=w507:dbl)  [unwired: 1 out]
                n395 = Multiply(x=w507, y=100.0) -> (x*y=w505:dbl)
                n396 = case shown="4" w505 {
                  frame 0, Default {
                  }
                  frame 1 {
                    n397 = local write "Score"(7.51 ("Numeric")) -> ()
                  }
                  frame 2 {
                    n398 = local write "Score"(7.52 ("Numeric")) -> ()
                  }
                  frame 3 {
                    n399 = local write "Score"(7.53 ("Numeric")) -> ()
                  }
                  frame 4 {
                    n400 = local write "Score"(7.54 ("Numeric")) -> ()
                  }
                }
              }
              frame 11 {
                n401 = Quotient & Remainder(x=w513, y=1.0) -> (x-y*floor(x/y)=w516:dbl)  [unwired: 1 out]
                n402 = Multiply(x=w516, y=100.0) -> (x*y=w514:dbl)
                n403 = case shown="4" w514 {
                  frame 0, Default {
                  }
                  frame 1 {
                    n404 = local write "Score"(7.41 ("Numeric")) -> ()
                  }
                  frame 2 {
                    n405 = local write "Score"(7.42 ("Numeric")) -> ()
                  }
                  frame 3 {
                    n406 = local write "Score"(7.43 ("Numeric")) -> ()
                  }
                  frame 4 {
                    n407 = local write "Score"(7.44 ("Numeric")) -> ()
                  }
                }
              }
              frame 12 {
                n408 = Quotient & Remainder(x=w522, y=1.0) -> (x-y*floor(x/y)=w525:dbl)  [unwired: 1 out]
                n409 = Multiply(x=w525, y=100.0) -> (x*y=w523:dbl)
                n410 = case shown="4" w523 {
                  frame 0, Default {
                  }
                  frame 1 {
                    n411 = local write "Score"(7.31 ("Numeric")) -> ()
                  }
                  frame 2 {
                    n412 = local write "Score"(7.32 ("Numeric")) -> ()
                  }
                  frame 3 {
                    n413 = local write "Score"(7.33 ("Numeric")) -> ()
                  }
                  frame 4 {
                    n414 = local write "Score"(7.34 ("Numeric")) -> ()
                  }
                }
              }
              frame 13 {
                n415 = Quotient & Remainder(x=w531, y=1.0) -> (x-y*floor(x/y)=w534:dbl)  [unwired: 1 out]
                n416 = Multiply(x=w534, y=100.0) -> (x*y=w532:dbl)
                n417 = case shown="4" w532 {
                  frame 0, Default {
                  }
                  frame 1 {
                    n418 = local write "Score"(7.21 ("Numeric")) -> ()
                  }
                  frame 2 {
                    n419 = local write "Score"(7.22 ("Numeric")) -> ()
                  }
                  frame 3 {
                    n420 = local write "Score"(7.23 ("Numeric")) -> ()
                  }
                  frame 4 {
                    n421 = local write "Score"(7.24 ("Numeric")) -> ()
                  }
                }
              }
            }
          }
          frame 8 {
            # "Two Pairs"
            n422 = Unbundle(w555) -> ("element"=w554:dbl, "element"=w553:dbl, "element"=w552:dbl, "element"=w551:dbl, "element"=w550:dbl)
            n423 = Build Array(w554, w553, w552, w551, w550) -> (w549:dbl[])
            n424 = Sort 1D Array(array=w549) -> (sorted array=w541:dbl[])
            n425 = Index Array(array=w541, index=1) -> (element=w542:dbl)
            n426 = Index Array(array=w541, index=3) -> (element=w540:dbl)
            n427 = Round Toward -Infinity(1:w542) -> (0:w543:dbl)
            n428 = Round Toward -Infinity(1:w540) -> (0:w544:dbl)
            n429 = Equal?(x=w543, y=1.0) -> (x = y?=w546:bool)
            n430 = case shown="5" w544 {
              tunnel: w540 -> [_ w556 w565 w574 w583 w592 w601 w610 w619 w628 w637 w646]
              frame 0, Default {
              }
              frame 3 {
                n431 = Quotient & Remainder(x=w556, y=1.0) -> (x-y*floor(x/y)=w558:dbl)  [unwired: 1 out]
                n432 = Multiply(x=w558, y=100.0) -> (x*y=w560:dbl)
                n433 = case shown="4" w560 {
                  frame 0, Default {
                  }
                  frame 1 {
                    n434 = local write "Score"(8.971 ("Numeric")) -> ()
                  }
                  frame 2 {
                    n435 = local write "Score"(8.972 ("Numeric")) -> ()
                  }
                  frame 3 {
                    n436 = local write "Score"(8.973 ("Numeric")) -> ()
                  }
                  frame 4 {
                    n437 = local write "Score"(8.974 ("Numeric")) -> ()
                  }
                }
              }
              frame 4 {
                n438 = Quotient & Remainder(x=w565, y=1.0) -> (x-y*floor(x/y)=w567:dbl)  [unwired: 1 out]
                n439 = Multiply(x=w567, y=100.0) -> (x*y=w569:dbl)
                n440 = case shown="3" w569 {
                  frame 0, Default {
                  }
                  frame 1 {
                    n441 = local write "Score"(8.961 ("Numeric")) -> ()
                  }
                  frame 2 {
                    n442 = local write "Score"(8.962 ("Numeric")) -> ()
                  }
                  frame 3 {
                    n443 = local write "Score"(8.963 ("Numeric")) -> ()
                  }
                  frame 4 {
                    n444 = local write "Score"(8.964 ("Numeric")) -> ()
                  }
                }
              }
              frame 5 {
                n445 = Quotient & Remainder(x=w574, y=1.0) -> (x-y*floor(x/y)=w576:dbl)  [unwired: 1 out]
                n446 = Multiply(x=w576, y=100.0) -> (x*y=w578:dbl)
                n447 = case shown="4" w578 {
                  frame 0, Default {
                  }
                  frame 1 {
                    n448 = local write "Score"(8.951 ("Numeric")) -> ()
                  }
                  frame 2 {
                    n449 = local write "Score"(8.952 ("Numeric")) -> ()
                  }
                  frame 3 {
                    n450 = local write "Score"(8.953 ("Numeric")) -> ()
                  }
                  frame 4 {
                    n451 = local write "Score"(8.954 ("Numeric")) -> ()
                  }
                }
              }
              frame 6 {
                n452 = Quotient & Remainder(x=w583, y=1.0) -> (x-y*floor(x/y)=w585:dbl)  [unwired: 1 out]
                n453 = Multiply(x=w585, y=100.0) -> (x*y=w587:dbl)
                n454 = case shown="4" w587 {
                  frame 0, Default {
                  }
                  frame 1 {
                    n455 = local write "Score"(8.91 ("Numeric")) -> ()
                  }
                  frame 2 {
                    n456 = local write "Score"(8.92 ("Numeric")) -> ()
                  }
                  frame 3 {
                    n457 = local write "Score"(8.93 ("Numeric")) -> ()
                  }
                  frame 4 {
                    n458 = local write "Score"(8.94 ("Numeric")) -> ()
                  }
                }
              }
              frame 7 {
                n459 = Quotient & Remainder(x=w592, y=1.0) -> (x-y*floor(x/y)=w594:dbl)  [unwired: 1 out]
                n460 = Multiply(x=w594, y=100.0) -> (x*y=w596:dbl)
                n461 = case shown="4" w596 {
                  frame 0, Default {
                  }
                  frame 1 {
                    n462 = local write "Score"(8.81 ("Numeric")) -> ()
                  }
                  frame 2 {
                    n463 = local write "Score"(8.82 ("Numeric")) -> ()
                  }
                  frame 3 {
                    n464 = local write "Score"(8.83 ("Numeric")) -> ()
                  }
                  frame 4 {
                    n465 = local write "Score"(8.84 ("Numeric")) -> ()
                  }
                }
              }
              frame 8 {
                n466 = Quotient & Remainder(x=w601, y=1.0) -> (x-y*floor(x/y)=w603:dbl)  [unwired: 1 out]
                n467 = Multiply(x=w603, y=100.0) -> (x*y=w605:dbl)
                n468 = case shown="4" w605 {
                  frame 0, Default {
                  }
                  frame 1 {
                    n469 = local write "Score"(8.71 ("Numeric")) -> ()
                  }
                  frame 2 {
                    n470 = local write "Score"(8.72 ("Numeric")) -> ()
                  }
                  frame 3 {
                    n471 = local write "Score"(8.73 ("Numeric")) -> ()
                  }
                  frame 4 {
                    n472 = local write "Score"(8.74 ("Numeric")) -> ()
                  }
                }
              }
              frame 9 {
                n473 = Quotient & Remainder(x=w610, y=1.0) -> (x-y*floor(x/y)=w612:dbl)  [unwired: 1 out]
                n474 = Multiply(x=w612, y=100.0) -> (x*y=w614:dbl)
                n475 = case shown="4" w614 {
                  frame 0, Default {
                  }
                  frame 1 {
                    n476 = local write "Score"(8.61 ("Numeric")) -> ()
                  }
                  frame 2 {
                    n477 = local write "Score"(8.62 ("Numeric")) -> ()
                  }
                  frame 3 {
                    n478 = local write "Score"(8.63 ("Numeric")) -> ()
                  }
                  frame 4 {
                    n479 = local write "Score"(8.64 ("Numeric")) -> ()
                  }
                }
              }
              frame 10 {
                n480 = Quotient & Remainder(x=w619, y=1.0) -> (x-y*floor(x/y)=w621:dbl)  [unwired: 1 out]
                n481 = Multiply(x=w621, y=100.0) -> (x*y=w623:dbl)
                n482 = case shown="4" w623 {
                  frame 0, Default {
                  }
                  frame 1 {
                    n483 = local write "Score"(8.51 ("Numeric")) -> ()
                  }
                  frame 2 {
                    n484 = local write "Score"(8.52 ("Numeric")) -> ()
                  }
                  frame 3 {
                    n485 = local write "Score"(8.53 ("Numeric")) -> ()
                  }
                  frame 4 {
                    n486 = local write "Score"(8.54 ("Numeric")) -> ()
                  }
                }
              }
              frame 11 {
                n487 = Quotient & Remainder(x=w628, y=1.0) -> (x-y*floor(x/y)=w630:dbl)  [unwired: 1 out]
                n488 = Multiply(x=w630, y=100.0) -> (x*y=w632:dbl)
                n489 = case shown="4" w632 {
                  frame 0, Default {
                  }
                  frame 1 {
                    n490 = local write "Score"(8.41 ("Numeric")) -> ()
                  }
                  frame 2 {
                    n491 = local write "Score"(8.42 ("Numeric")) -> ()
                  }
                  frame 3 {
                    n492 = local write "Score"(8.43 ("Numeric")) -> ()
                  }
                  frame 4 {
                    n493 = local write "Score"(8.44 ("Numeric")) -> ()
                  }
                }
              }
              frame 12 {
                n494 = Quotient & Remainder(x=w637, y=1.0) -> (x-y*floor(x/y)=w639:dbl)  [unwired: 1 out]
                n495 = Multiply(x=w639, y=100.0) -> (x*y=w641:dbl)
                n496 = case shown="4" w641 {
                  frame 0, Default {
                  }
                  frame 1 {
                    n497 = local write "Score"(8.31 ("Numeric")) -> ()
                  }
                  frame 2 {
                    n498 = local write "Score"(8.32 ("Numeric")) -> ()
                  }
                  frame 3 {
                    n499 = local write "Score"(8.33 ("Numeric")) -> ()
                  }
                  frame 4 {
                    n500 = local write "Score"(8.34 ("Numeric")) -> ()
                  }
                }
              }
              frame 13 {
                n501 = Quotient & Remainder(x=w646, y=1.0) -> (x-y*floor(x/y)=w648:dbl)  [unwired: 1 out]
                n502 = Multiply(x=w648, y=100.0) -> (x*y=w650:dbl)
                n503 = case shown="1" w650 {
                  frame 0, Default {
                  }
                  frame 1 {
                    n504 = local write "Score"(8.21 ("Numeric")) -> ()
                  }
                  frame 2 {
                    n505 = local write "Score"(8.22 ("Numeric")) -> ()
                  }
                  frame 3 {
                    n506 = local write "Score"(8.23 ("Numeric")) -> ()
                  }
                  frame 4 {
                    n507 = local write "Score"(8.24 ("Numeric")) -> ()
                  }
                }
              }
            }
            n508 = case shown="True" w546 {
              tunnel: w542 -> [_ w655]
              frame False {
              }
              frame True {
                n509 = Quotient & Remainder(x=w655, y=1.0) -> (x-y*floor(x/y)=w658:dbl)  [unwired: 1 out]
                n510 = Multiply(x=w658, y=100.0) -> (x*y=w656:dbl)
                n511 = case shown="1" w656 {
                  frame 0, Default {
                  }
                  frame 1 {
                    n512 = local write "Score"(8.11 ("Numeric")) -> ()
                  }
                  frame 2 {
                    n513 = local write "Score"(8.12 ("Numeric")) -> ()
                  }
                  frame 3 {
                    n514 = local write "Score"(8.13 ("Numeric")) -> ()
                  }
                  frame 4 {
                    n515 = local write "Score"(8.14 ("Numeric")) -> ()
                  }
                }
              }
            }
          }
          frame 9 {
            n516 = flat-sequence {
              tunnel: w664 -> [w679]
              frame #0 {
                # "One pair"
                n517 = Unbundle(w679) -> ("element"=w668:dbl, "element"=w667:dbl, "element"=w666:dbl, "element"=w665:dbl, "element"=w671:dbl)
                n518 = Round Toward -Infinity(1:w671) -> (0:w670:dbl)
                n519 = Round Toward -Infinity(1:w668) -> (0:w674:dbl)
                n520 = Round Toward -Infinity(1:w667) -> (0:w673:dbl)
                n521 = Round Toward -Infinity(1:w665) -> (0:w669:dbl)
                n522 = Round Toward -Infinity(1:w666) -> (0:w672:dbl)
                n523 = Equal?(x=w674, y=w673) -> (x = y?=w678:bool)
                n524 = Equal?(x=w673, y=w672) -> (x = y?=w677:bool)
                n525 = Equal?(x=w672, y=w669) -> (x = y?=w676:bool)
                n526 = Equal?(x=w669, y=w670) -> (x = y?=w675:bool)
                n527 = case shown="True" w675 {
                  tunnel: w669 -> [_ w681]
                  tunnel: w665 -> [_ w680]
                  frame False {
                  }
                  frame True {
                    n528 = local write "Pair's value"(w681) -> ()
                    n529 = local write "Pair's DBL"(w680) -> ()
                  }
                }
                n530 = case shown="True" w676 {
                  tunnel: w672 -> [_ w683]
                  tunnel: w666 -> [_ w682]
                  frame False {
                  }
                  frame True {
                    n531 = local write "Pair's value"(w683) -> ()
                    n532 = local write "Pair's DBL"(w682) -> ()
                  }
                }
                n533 = case shown="True" w677 {
                  tunnel: w673 -> [_ w685]
                  tunnel: w667 -> [_ w684]
                  frame False {
                  }
                  frame True {
                    n534 = local write "Pair's value"(w685) -> ()
                    n535 = local write "Pair's DBL"(w684) -> ()
                  }
                }
                n536 = case shown="True" w678 {
                  tunnel: w674 -> [_ w687]
                  tunnel: w668 -> [_ w686]
                  frame False {
                  }
                  frame True {
                    n537 = local write "Pair's value"(w687) -> ()
                    n538 = local write "Pair's DBL"(w686) -> ()
                  }
                }
              }
              frame #1 {
                n539 = case shown="5" "Pair's value" {
                  tunnel: "Pair's DBL" -> [_ w690 w699 w709 w718 w727 w736 w745 w754 w763 w772 w781 w790 w799]
                  frame 0, Default {
                  }
                  frame 1 {
                    n540 = Quotient & Remainder(x=w690, y=1.0) -> (x-y*floor(x/y)=w692:dbl)  [unwired: 1 out]
                    n541 = Multiply(x=w692, y=100.0) -> (x*y=w694:dbl)
                    n542 = case shown="4" w694 {
                      frame 0, Default {
                      }
                      frame 1 {
                        n543 = local write "Score"(9.11 ("Numeric")) -> ()
                      }
                      frame 2 {
                        n544 = local write "Score"(9.12 ("Numeric")) -> ()
                      }
                      frame 3 {
                        n545 = local write "Score"(9.13 ("Numeric")) -> ()
                      }
                      frame 4 {
                        n546 = local write "Score"(9.14 ("Numeric")) -> ()
                      }
                    }
                  }
                  frame 2 {
                    n547 = Quotient & Remainder(x=w699, y=1.0) -> (x-y*floor(x/y)=w701:dbl)  [unwired: 1 out]
                    n548 = Multiply(x=w701, y=100.0) -> (x*y=w703:dbl)
                    n549 = case shown="4" w703 {
                      frame 0, Default {
                      }
                      frame 1 {
                        n550 = local write "Score"(9.981 ("Numeric")) -> ()
                      }
                      frame 2 {
                        n551 = local write "Score"(9.982 ("Numeric")) -> ()
                      }
                      frame 3 {
                        n552 = local write "Score"(9.983 ("Numeric")) -> ()
                      }
                      frame 4 {
                        n553 = local write "Score"(9.984 ("Numeric")) -> ()
                      }
                    }
                    n554 = local write "Score"(7.94 ("Numeric")) -> ()
                  }
                  frame 3 {
                    n555 = Quotient & Remainder(x=w709, y=1.0) -> (x-y*floor(x/y)=w711:dbl)  [unwired: 1 out]
                    n556 = Multiply(x=w711, y=100.0) -> (x*y=w713:dbl)
                    n557 = case shown="4" w713 {
                      frame 0, Default {
                      }
                      frame 1 {
                        n558 = local write "Score"(9.971 ("Numeric")) -> ()
                      }
                      frame 2 {
                        n559 = local write "Score"(9.972 ("Numeric")) -> ()
                      }
                      frame 3 {
                        n560 = local write "Score"(9.973 ("Numeric")) -> ()
                      }
                      frame 4 {
                        n561 = local write "Score"(9.974 ("Numeric")) -> ()
                      }
                    }
                  }
                  frame 4 {
                    n562 = Quotient & Remainder(x=w718, y=1.0) -> (x-y*floor(x/y)=w720:dbl)  [unwired: 1 out]
                    n563 = Multiply(x=w720, y=100.0) -> (x*y=w722:dbl)
                    n564 = case shown="1" w722 {
                      frame 0, Default {
                      }
                      frame 1 {
                        n565 = local write "Score"(9.961 ("Numeric")) -> ()
                      }
                      frame 2 {
                        n566 = local write "Score"(9.962 ("Numeric")) -> ()
                      }
                      frame 3 {
                        n567 = local write "Score"(9.963 ("Numeric")) -> ()
                      }
                      frame 4 {
                        n568 = local write "Score"(9.964 ("Numeric")) -> ()
                      }
                    }
                  }
                  frame 5 {
                    n569 = Quotient & Remainder(x=w727, y=1.0) -> (x-y*floor(x/y)=w729:dbl)  [unwired: 1 out]
                    n570 = Multiply(x=w729, y=100.0) -> (x*y=w731:dbl)
                    n571 = case shown="4" w731 {
                      frame 0, Default {
                      }
                      frame 1 {
                        n572 = local write "Score"(9.951 ("Numeric")) -> ()
                      }
                      frame 2 {
                        n573 = local write "Score"(9.952 ("Numeric")) -> ()
                      }
                      frame 3 {
                        n574 = local write "Score"(9.953 ("Numeric")) -> ()
                      }
                      frame 4 {
                        n575 = local write "Score"(9.954 ("Numeric")) -> ()
                      }
                    }
                  }
                  frame 6 {
                    n576 = Quotient & Remainder(x=w736, y=1.0) -> (x-y*floor(x/y)=w738:dbl)  [unwired: 1 out]
                    n577 = Multiply(x=w738, y=100.0) -> (x*y=w740:dbl)
                    n578 = case shown="4" w740 {
                      frame 0, Default {
                      }
                      frame 1 {
                        n579 = local write "Score"(9.91 ("Numeric")) -> ()
                      }
                      frame 2 {
                        n580 = local write "Score"(9.92 ("Numeric")) -> ()
                      }
                      frame 3 {
                        n581 = local write "Score"(9.93 ("Numeric")) -> ()
                      }
                      frame 4 {
                        n582 = local write "Score"(9.94 ("Numeric")) -> ()
                      }
                    }
                  }
                  frame 7 {
                    n583 = Quotient & Remainder(x=w745, y=1.0) -> (x-y*floor(x/y)=w747:dbl)  [unwired: 1 out]
                    n584 = Multiply(x=w747, y=100.0) -> (x*y=w749:dbl)
                    n585 = case shown="4" w749 {
                      frame 0, Default {
                      }
                      frame 1 {
                        n586 = local write "Score"(9.81 ("Numeric")) -> ()
                      }
                      frame 2 {
                        n587 = local write "Score"(9.82 ("Numeric")) -> ()
                      }
                      frame 3 {
                        n588 = local write "Score"(9.83 ("Numeric")) -> ()
                      }
                      frame 4 {
                        n589 = local write "Score"(9.84 ("Numeric")) -> ()
                      }
                    }
                  }
                  frame 8 {
                    n590 = Quotient & Remainder(x=w754, y=1.0) -> (x-y*floor(x/y)=w756:dbl)  [unwired: 1 out]
                    n591 = Multiply(x=w756, y=100.0) -> (x*y=w758:dbl)
                    n592 = case shown="4" w758 {
                      frame 0, Default {
                      }
                      frame 1 {
                        n593 = local write "Score"(9.71 ("Numeric")) -> ()
                      }
                      frame 2 {
                        n594 = local write "Score"(9.72 ("Numeric")) -> ()
                      }
                      frame 3 {
                        n595 = local write "Score"(9.73 ("Numeric")) -> ()
                      }
                      frame 4 {
                        n596 = local write "Score"(9.74 ("Numeric")) -> ()
                      }
                    }
                  }
                  frame 9 {
                    n597 = Quotient & Remainder(x=w763, y=1.0) -> (x-y*floor(x/y)=w765:dbl)  [unwired: 1 out]
                    n598 = Multiply(x=w765, y=100.0) -> (x*y=w767:dbl)
                    n599 = case shown="4" w767 {
                      frame 0, Default {
                      }
                      frame 1 {
                        n600 = local write "Score"(9.61 ("Numeric")) -> ()
                      }
                      frame 2 {
                        n601 = local write "Score"(9.62 ("Numeric")) -> ()
                      }
                      frame 3 {
                        n602 = local write "Score"(9.63 ("Numeric")) -> ()
                      }
                      frame 4 {
                        n603 = local write "Score"(9.64 ("Numeric")) -> ()
                      }
                    }
                  }
                  frame 10 {
                    n604 = Quotient & Remainder(x=w772, y=1.0) -> (x-y*floor(x/y)=w774:dbl)  [unwired: 1 out]
                    n605 = Multiply(x=w774, y=100.0) -> (x*y=w776:dbl)
                    n606 = case shown="4" w776 {
                      frame 0, Default {
                      }
                      frame 1 {
                        n607 = local write "Score"(9.51 ("Numeric")) -> ()
                      }
                      frame 2 {
                        n608 = local write "Score"(9.52 ("Numeric")) -> ()
                      }
                      frame 3 {
                        n609 = local write "Score"(9.53 ("Numeric")) -> ()
                      }
                      frame 4 {
                        n610 = local write "Score"(9.54 ("Numeric")) -> ()
                      }
                    }
                  }
                  frame 11 {
                    n611 = Quotient & Remainder(x=w781, y=1.0) -> (x-y*floor(x/y)=w783:dbl)  [unwired: 1 out]
                    n612 = Multiply(x=w783, y=100.0) -> (x*y=w785:dbl)
                    n613 = case shown="4" w785 {
                      frame 0, Default {
                      }
                      frame 1 {
                        n614 = local write "Score"(9.41 ("Numeric")) -> ()
                      }
                      frame 2 {
                        n615 = local write "Score"(9.42 ("Numeric")) -> ()
                      }
                      frame 3 {
                        n616 = local write "Score"(9.43 ("Numeric")) -> ()
                      }
                      frame 4 {
                        n617 = local write "Score"(9.44 ("Numeric")) -> ()
                      }
                    }
                  }
                  frame 12 {
                    n618 = Quotient & Remainder(x=w790, y=1.0) -> (x-y*floor(x/y)=w792:dbl)  [unwired: 1 out]
                    n619 = Multiply(x=w792, y=100.0) -> (x*y=w794:dbl)
                    n620 = case shown="4" w794 {
                      frame 0, Default {
                      }
                      frame 1 {
                        n621 = local write "Score"(9.31 ("Numeric")) -> ()
                      }
                      frame 2 {
                        n622 = local write "Score"(9.32 ("Numeric")) -> ()
                      }
                      frame 3 {
                        n623 = local write "Score"(9.33 ("Numeric")) -> ()
                      }
                      frame 4 {
                        n624 = local write "Score"(9.34 ("Numeric")) -> ()
                      }
                    }
                  }
                  frame 13 {
                    n625 = Quotient & Remainder(x=w799, y=1.0) -> (x-y*floor(x/y)=w801:dbl)  [unwired: 1 out]
                    n626 = Multiply(x=w801, y=100.0) -> (x*y=w803:dbl)
                    n627 = case shown="4" w803 {
                      frame 0, Default {
                      }
                      frame 1 {
                        n628 = local write "Score"(9.21 ("Numeric")) -> ()
                      }
                      frame 2 {
                        n629 = local write "Score"(9.22 ("Numeric")) -> ()
                      }
                      frame 3 {
                        n630 = local write "Score"(9.23 ("Numeric")) -> ()
                      }
                      frame 4 {
                        n631 = local write "Score"(9.24 ("Numeric")) -> ()
                      }
                    }
                  }
                }
              }
            }
          }
          frame 10 {
            # "High Card"
            n632 = Unbundle(w808) -> ("element"=w810:dbl, "element"=w809:dbl)  [unwired: 3 out]
            n633 = Round Toward -Infinity(1:w810) -> (0:w814:dbl)
            n634 = Round Toward -Infinity(1:w809) -> (0:w811:dbl)
            n635 = Equal?(x=w814, y=1.0) -> (x = y?=w813:bool)
            n636 = case shown="7" w811 {
              tunnel: w809 -> [_ w815 w824 w833 w842 w851 w860 w869]
              frame 0, Default {
              }
              frame 7 {
                n637 = Quotient & Remainder(x=w815, y=1.0) -> (x-y*floor(x/y)=w818:dbl)  [unwired: 1 out]
                n638 = Multiply(x=w818, y=100.0) -> (x*y=w816:dbl)
                n639 = case shown="3" w816 {
                  frame 0, Default {
                  }
                  frame 1 {
                    n640 = local write "Score"(10.81 ("Numeric")) -> ()
                  }
                  frame 2 {
                    n641 = local write "Score"(10.82 ("Numeric")) -> ()
                  }
                  frame 3 {
                    n642 = local write "Score"(10.83 ("Numeric")) -> ()
                  }
                  frame 4 {
                    n643 = local write "Score"(10.84 ("Numeric")) -> ()
                  }
                }
              }
              frame 8 {
                n644 = Quotient & Remainder(x=w824, y=1.0) -> (x-y*floor(x/y)=w827:dbl)  [unwired: 1 out]
                n645 = Multiply(x=w827, y=100.0) -> (x*y=w825:dbl)
                n646 = case shown="4" w825 {
                  frame 0, Default {
                  }
                  frame 1 {
                    n647 = local write "Score"(10.71 ("Numeric")) -> ()
                  }
                  frame 2 {
                    n648 = local write "Score"(10.72 ("Numeric")) -> ()
                  }
                  frame 3 {
                    n649 = local write "Score"(10.73 ("Numeric")) -> ()
                  }
                  frame 4 {
                    n650 = local write "Score"(10.74 ("Numeric")) -> ()
                  }
                }
              }
              frame 9 {
                n651 = Quotient & Remainder(x=w833, y=1.0) -> (x-y*floor(x/y)=w836:dbl)  [unwired: 1 out]
                n652 = Multiply(x=w836, y=100.0) -> (x*y=w834:dbl)
                n653 = case shown="1" w834 {
                  frame 0, Default {
                  }
                  frame 1 {
                    n654 = local write "Score"(10.61 ("Numeric")) -> ()
                  }
                  frame 2 {
                    n655 = local write "Score"(10.62 ("Numeric")) -> ()
                  }
                  frame 3 {
                    n656 = local write "Score"(10.63 ("Numeric")) -> ()
                  }
                  frame 4 {
                    n657 = local write "Score"(10.64 ("Numeric")) -> ()
                  }
                }
              }
              frame 10 {
                n658 = Quotient & Remainder(x=w842, y=1.0) -> (x-y*floor(x/y)=w845:dbl)  [unwired: 1 out]
                n659 = Multiply(x=w845, y=100.0) -> (x*y=w843:dbl)
                n660 = case shown="4" w843 {
                  frame 0, Default {
                  }
                  frame 1 {
                    n661 = local write "Score"(10.51 ("Numeric")) -> ()
                  }
                  frame 2 {
                    n662 = local write "Score"(10.52 ("Numeric")) -> ()
                  }
                  frame 3 {
                    n663 = local write "Score"(10.53 ("Numeric")) -> ()
                  }
                  frame 4 {
                    n664 = local write "Score"(10.54 ("Numeric")) -> ()
                  }
                }
              }
              frame 11 {
                n665 = Quotient & Remainder(x=w851, y=1.0) -> (x-y*floor(x/y)=w854:dbl)  [unwired: 1 out]
                n666 = Multiply(x=w854, y=100.0) -> (x*y=w852:dbl)
                n667 = case shown="4" w852 {
                  frame 0, Default {
                  }
                  frame 1 {
                    n668 = local write "Score"(10.41 ("Numeric")) -> ()
                  }
                  frame 2 {
                    n669 = local write "Score"(10.42 ("Numeric")) -> ()
                  }
                  frame 3 {
                    n670 = local write "Score"(10.43 ("Numeric")) -> ()
                  }
                  frame 4 {
                    n671 = local write "Score"(10.44 ("Numeric")) -> ()
                  }
                }
              }
              frame 12 {
                n672 = Quotient & Remainder(x=w860, y=1.0) -> (x-y*floor(x/y)=w863:dbl)  [unwired: 1 out]
                n673 = Multiply(x=w863, y=100.0) -> (x*y=w861:dbl)
                n674 = case shown="4" w861 {
                  frame 0, Default {
                  }
                  frame 1 {
                    n675 = local write "Score"(10.31 ("Numeric")) -> ()
                  }
                  frame 2 {
                    n676 = local write "Score"(10.32 ("Numeric")) -> ()
                  }
                  frame 3 {
                    n677 = local write "Score"(10.33 ("Numeric")) -> ()
                  }
                  frame 4 {
                    n678 = local write "Score"(10.34 ("Numeric")) -> ()
                  }
                }
              }
              frame 13 {
                n679 = Quotient & Remainder(x=w869, y=1.0) -> (x-y*floor(x/y)=w872:dbl)  [unwired: 1 out]
                n680 = Multiply(x=w872, y=100.0) -> (x*y=w870:dbl)
                n681 = case shown="4" w870 {
                  frame 0, Default {
                  }
                  frame 1 {
                    n682 = local write "Score"(10.21 ("Numeric")) -> ()
                  }
                  frame 2 {
                    n683 = local write "Score"(10.22 ("Numeric")) -> ()
                  }
                  frame 3 {
                    n684 = local write "Score"(10.23 ("Numeric")) -> ()
                  }
                  frame 4 {
                    n685 = local write "Score"(10.24 ("Numeric")) -> ()
                  }
                }
              }
            }
            n686 = case shown="True" w813 {
              tunnel: w810 -> [_ w878]
              frame False {
              }
              frame True {
                n687 = Quotient & Remainder(x=w878, y=1.0) -> (x-y*floor(x/y)=w881:dbl)  [unwired: 1 out]
                n688 = Multiply(x=w881, y=100.0) -> (x*y=w879:dbl)
                n689 = case shown="4" w879 {
                  frame 0, Default {
                  }
                  frame 1 {
                    n690 = local write "Score"(10.11 ("Numeric")) -> ()
                  }
                  frame 2 {
                    n691 = local write "Score"(10.12 ("Numeric")) -> ()
                  }
                  frame 3 {
                    n692 = local write "Score"(10.13 ("Numeric")) -> ()
                  }
                  frame 4 {
                    n693 = local write "Score"(10.14 ("Numeric")) -> ()
                  }
                }
              }
            }
          }
        }
      }
      frame #1 {
        n694 = local read "Score"() -> (w889:dbl)
        n695 = Bundle("Score"=w889, w888) -> (w887:T4)  [unwired: 1 in]
      }
    }
  }
  n696 = Sort 1D Array(array=w2) -> (sorted array=→"Poker Hands Score and Combination":T1)
